vi "Convert to Previous version of LabVIEW.vi"(6 "Error Handling":T1(ring), 7 "Previous Version":string(combo)="9.0", 8 "error in (no error)":errorcluster, 10 "Destination for down converted files.":path, 11 "Folder of LabVIEW files":path) -> (0 "error out":errorcluster, 3 "Path out":path)   [LabVIEW 2023]
doc: "This VI will convert a folder of VIs to a previous (selectable) version of LabVIEW."
uses:
  <userlib>/_OpenG.lib/file/file.llb/Strip Path Extension - Path__ogtk.vi
panel:
  out "ALL Errors":errorcluster[](array[cluster])
  out "Path":path
  out "Progress":string
  # "Overview:This VI will convert a folder of VIs to a previous (selectable) version of LabVIEW.\nRequirements: LabVIEW 2012 or compatible\nInstructions:\n1.choose the Previous Version\n2.Run VI"
  # "Mass Compile for previous version"
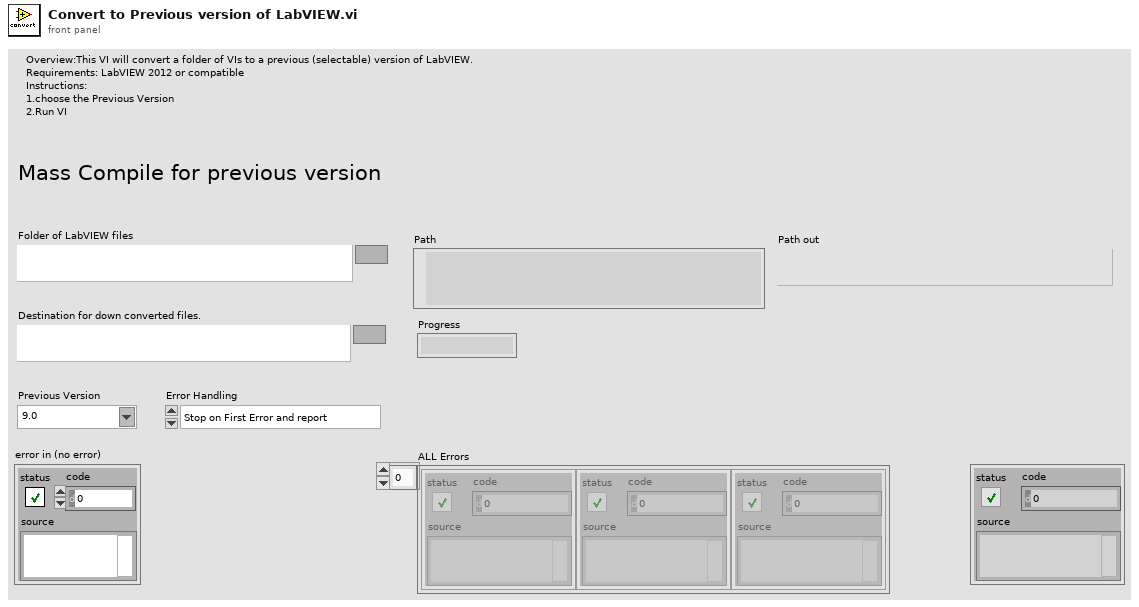
[diagram p1: front panel]
types:
  T1 = enum16{"Stop on First Error and report", "Continue on Error and Report", "Clear all Errors"}
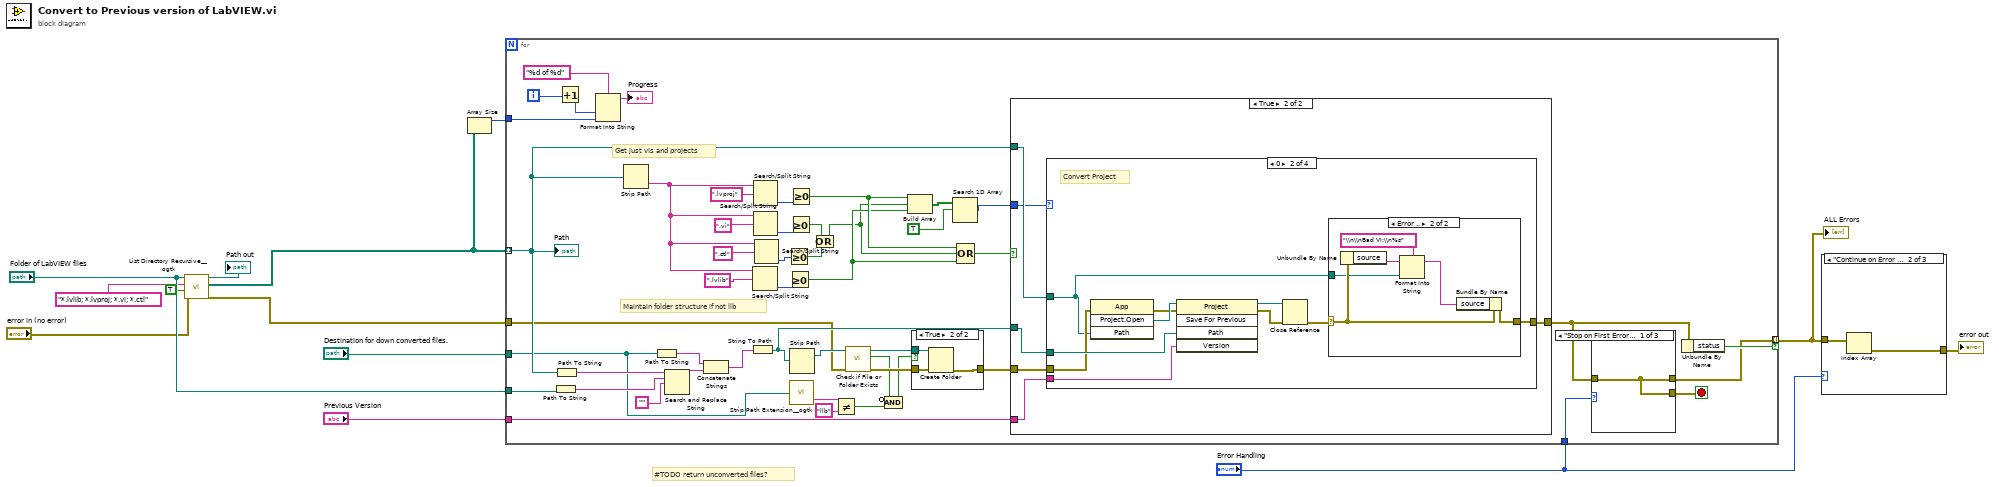
[diagram p0: block diagram]
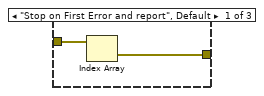
[diagram p2: hidden frame]
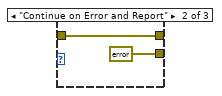
[diagram p4: hidden frame]
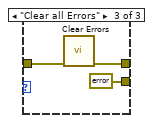
[diagram p5: hidden frame]
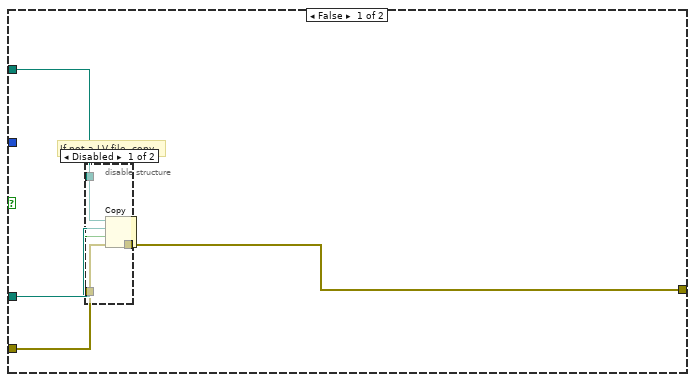
[diagram p6: hidden frame]
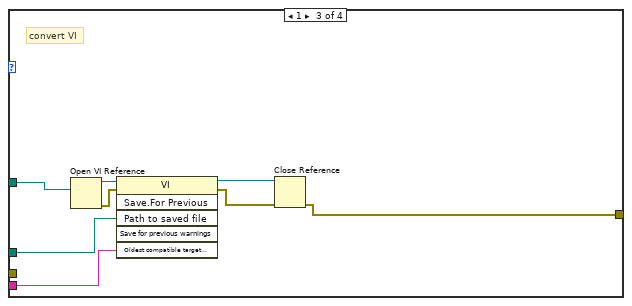
[diagram p10: hidden frame]
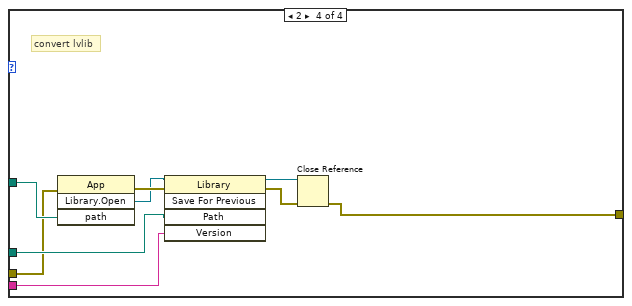
[diagram p11: hidden frame]
diagram:
  # "#TODO return unconverted files?"
  n1 = call <userlib>:"List Directory Recursive__ogtk.vi"("error in (no error)"="error in (no error)", "Treat llb files as directories? (FALSE)"=TRUE, "pattern"="*.lvlib; *.lvproj; *.vi; *.ctl", "Path"="Folder of LabVIEW files") -> ("error out"=w4:errorcluster, "file paths"=w9:path[], "dup Path"=→"Path out":path)  [unwired: 4 in, 1 out]
  n2 = Array Size(array=w9) -> (size(s)=w11:i32)
  n3 = for {
    tunnel: w9 -> [w49] mode=indexing
    tunnel: "Destination for down converted files." -> [w31]
    tunnel: "Folder of LabVIEW files" -> [w62]
    tunnel: "Previous Version" -> [w54]
    tunnel: w11 -> [w46]
    tunnel: [w17] -> w3 mode=indexing if=w18
    tunnel: "Error Handling" -> [w19]
    tunnel: w4 -> [w15]
    i -> [w48]
    stop <- w14 stop-if-true
    # "Get just vis and projects"
    # "Maintain folder structure if not llb"
    n4 = Path To String(path=w62) -> (string=w60:string)
    n5 = Path To String(path=w49) -> (string=w61:string)
    n6 = Increment(x=w48) -> (x+1=w47:i32)
    n7 = Format Into String(format string="%d of %d" ("search string"), w47, w46) -> (resulting string=→"Progress":string)  [unwired: 2 in, 1 out]
    n8 = Strip Path(path=w49) -> (name=w25:string)  [unwired: 1 out]
    n9 = Path To String(path=w31) -> (string=w58:string)
    n10 = Search and Replace String(input string=w61, search string=w60, replace string="") -> (result string=w57:string)  [unwired: 5 in, 3 out]
    n11 = Concatenate Strings(w58, w57) -> (w56:string)
    n12 = String To Path(string=w56) -> (path=w55:path)
    n13 = Search/Split String(string=w25, search string/char (-)=".lvlib" ("search string")) -> (offset of match=w34:i32)  [unwired: 1 in, 2 out]
    n14 = Search/Split String(string=w25, search string/char (-)=".lvproj" ("search string")) -> (offset of match=w36:i32)  [unwired: 1 in, 2 out]
    n15 = Search/Split String(string=w25, search string/char (-)=".vi" ("search string")) -> (offset of match=w32:i32)  [unwired: 1 in, 2 out]
    n16 = Search/Split String(string=w25, search string/char (-)=".ctl" ("search string")) -> (offset of match=w23:i32)  [unwired: 1 in, 2 out]
    n17 = Greater Or Equal To 0?(x=w23) -> (x >= 0?=w22:bool)
    n18 = Greater Or Equal To 0?(x=w34) -> (x >= 0?=w41:bool)
    n19 = Greater Or Equal To 0?(x=w32) -> (x >= 0?=w21:bool)
    n20 = Greater Or Equal To 0?(x=w36) -> (x >= 0?=w42:bool)
    n21 = call-poly <userlib>:"Strip Path Extension__ogtk.vi"("path"=w31) -> ("extension"=w30:string)  [unwired: 1 out]
    n22 = Strip Path(path=w55) -> (stripped path=w52:path)  [unwired: 1 out]
    n23 = Or(x=w21, y=w22) -> (x .or. y?=w20:bool)
    n24 = Not Equal?(x=w30, y="llb") -> (x != y?=w28:bool)
    n25 = call <vilib>:"Check if File or Folder Exists.vi"("error in (no error)"=w15, "path"=w52) -> ("error out"=w51:errorcluster, "file or folder exists?"=w27:bool, "dup path"=w43:path)  [unwired: 7 in]
    n26 = Compound Arithmetic op=AND(invert w27, w28) -> (w26:bool)
    n27 = Build Array(w42, w20, w41) -> (w40:bool[])
    n28 = case shown="True" w26 {
      tunnel: [w119 w122] -> w53
      tunnel: w51 -> [w119 w121]
      tunnel: w43 -> [_ w120]
      frame False {
      }
      frame True {
        n29 = Create Folder(path (use dialog)=w120, error in=w121) -> (error out=w122:errorcluster)  [unwired: 1 in, 2 out]
      }
    }
    n30 = Search 1D Array(1D array=w40, element=TRUE ("x >= 0?")) -> (index of element=w38:i32)  [unwired: 1 in]
    n31 = Compound Arithmetic op=OR(w42, w20, w41) -> (w50:bool)
    n32 = case shown="True" w50 {
      tunnel: [w69 w83] -> w16
      tunnel: w55 -> [w71 w79]
      tunnel: w54 -> [_ w82]
      tunnel: w53 -> [w70 w81]
      tunnel: w49 -> [w72 w80]
      tunnel: w38 -> [_ w78]
      frame False {
        # "If not a LV file, copy"
        n33 = disable-structure shown="Disabled" {
          disable-tunnel: w72 -> [w77 _]
          disable-tunnel: w71 -> [w76 _]
          disable-tunnel: w70 -> [w75 _]
          disable-tunnel: [w73 _] -> w69
          frame Disabled {
            n34 = Copy(8:w75, 9:TRUE ("overwrite (F)"), 10:w76, 11:w77) -> (0:w73:errorcluster)  [unwired: 1 in, 2 out]
          }
          frame Enabled {
          }
        }
      }
      frame True {
        n35 = case shown="0" w78 {
          tunnel: w79 -> [_ w91 w108 w114]
          tunnel: w80 -> [_ w85 w106 w116]
          tunnel: [w84 w86 w103 w112] -> w83
          tunnel: w82 -> [_ w89 w102 w113]
          tunnel: w81 -> [w84 w88 _ w111]
          frame -1, Default {
          }
          frame 0 {
            # "Convert Project"
            n36 = invoke class="App" method="Project.Open"(error in=w88, "Path"=w85) -> (error out=w92:errorcluster, "Project:Open"=w94:refnum<vi>)  [unwired: 2 in, 2 out]
            n37 = invoke class="Project" method="Save For Previous"(reference=w94, error in=w92, "Path"=w91, "Version"=w89) -> (reference out=w93:refnum<vi>, error out=w90:errorcluster)  [unwired: 1 in, 3 out]
            n38 = Close Reference(reference=w93, error in (no error)=w90) -> (error out=w87:errorcluster)
            n39 = case shown="Error .." w87 {
              selector: w87 -> [w95 w101]
              tunnel: [w95 w100] -> w86
              tunnel: w85 -> [_ w98]
              frame No Error {
              }
              frame Error {
                n40 = Unbundle By Name(w101) -> ("source"=w99:string)
                n41 = Format Into String(format string="\\n\\nBad VI:\\n%s", initial string=w99, w98) -> (resulting string=w96:string)  [unwired: 1 in, 1 out]
                n42 = Bundle By Name(cluster=w101, "source"=w96) -> (w100:errorcluster)
              }
            }
          }
          frame 1 {
            # "convert VI"
            n43 = Open VI Reference(vi path=w106) -> (vi reference=w107:refnum<vi>, error out=w109:errorcluster)  [unwired: 5 in]
            n44 = invoke class="VI" method="Save.For Previous"(reference=w107, error in=w109, "Path to saved file"=w108, "Oldest compatible target version"=w102) -> (reference out=w105:refnum<vi>, error out=w104:errorcluster)  [unwired: 2 in, 4 out]
            n45 = Close Reference(reference=w105, error in (no error)=w104) -> (error out=w103:errorcluster)
          }
          frame 2 {
            # "convert lvlib"
            n46 = invoke class="App" method="Library.Open"(error in=w111, "path"=w116) -> (error out=w118:errorcluster, "Open Library"=w115:refnum<vi>)  [unwired: 2 in, 2 out]
            n47 = invoke class="Library" method="Save For Previous"(reference=w115, error in=w118, "Path"=w114, "Version"=w113) -> (reference out=w110:refnum<vi>, error out=w117:errorcluster)  [unwired: 1 in, 3 out]
            n48 = Close Reference(reference=w110, error in (no error)=w117) -> (error out=w112:errorcluster)
          }
        }
      }
    }
    n49 = case shown="\"Stop on First Error and report\", Default" w19 {
      tunnel: [w63 w65 w67] -> w17
      tunnel: w16 -> [w63 w65 w68]
      tunnel: [w63 errorcluster {"status"=FALSE, "code"=0, "source"=""} ("error out") errorcluster {"status"=FALSE, "code"=0, "source"=""} ("error out")] -> w14
      frame "Stop on First Error and report", Default {
      }
      frame "Continue on Error and Report" {
      }
      frame "Clear all Errors" {
        n50 = call <vilib>:"Clear Errors.vi"("error in (no error)"=w68) -> ("error out"=w67:errorcluster)  [unwired: 5 in, 1 out]
      }
    }
    n51 = Unbundle By Name(w16) -> ("status"=w18:bool)
    "Path" <- w49
  }
  "ALL Errors" <- w3
  n52 = case shown="\"Continue on Error and Report\"" "Error Handling" {
    tunnel: w3 -> [w124 w125 _]
    tunnel: [w123 w126 _] -> w2
    frame "Stop on First Error and report", Default {
      n53 = Index Array(array=w124) -> (element=w123:errorcluster)  [unwired: 1 in]
    }
    frame "Continue on Error and Report" {
      n54 = Index Array(array=w125) -> (element=w126:errorcluster)  [unwired: 1 in]
    }
    frame "Clear all Errors" {
    }
  }
  "error out" <- w2
